vi "全局 1.vi"() -> ()   [LabVIEW 2013]
panel:
  out "通讯":bool
  out "状态号":i32
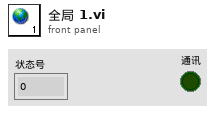
[diagram p1: front panel]
diagram:
